vi "sv_Convert Array of Peaks to XY Format.vi"(4 "peaks":cluster{"frequency [Hz]":dbl, "amplitude":dbl}[](array[cluster]) {"amplitude" format="%.2f"; "frequency [Hz]" format="%.2f"}) -> (1 "peaks":cluster{"X":dbl[], "Y":dbl[]} {"Y" format="%.2f"; "X" format="%.2f"})   [LabVIEW 2017]
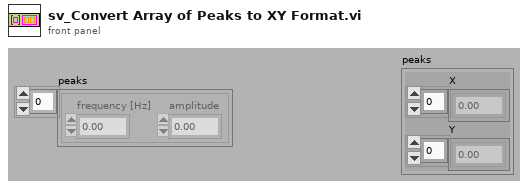
[diagram p1: front panel]
types:
  T1 = cluster{"frequencies [Hz]":dbl[], "values":dbl[]}
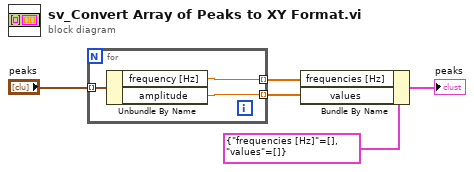
[diagram p0: block diagram]
diagram:
  n1 = for {
    tunnel: "peaks" -> [w8] mode=indexing
    tunnel: [w6] -> w2 mode=indexing
    tunnel: [w7] -> w3 mode=indexing
    n2 = Unbundle By Name(w8) -> ("frequency [Hz]"=w6:dbl, "amplitude"=w7:dbl)
  }
  n3 = Bundle By Name(cluster=T1 {"frequencies [Hz]"=[], "values"=[]} ("lower limit 2"), "frequencies [Hz]"=w2, "values"=w3) -> (→"peaks":T1)
